vi "Write Element of Coefficients.vi"(8 "error in (no error)":errorcluster, 9 "Numeric":dbl, 10 "index":i32, 11 "Thruster in":refnum<class "Thruster.lvclass">) -> (0 "error out":errorcluster, 3 "Thruster out":refnum<class "Thruster.lvclass">)   [LabVIEW 2014, in "Thruster.lvclass"]
uses:
  Thruster.lvclass
  Thruster.lvclass/Thruster.ctl
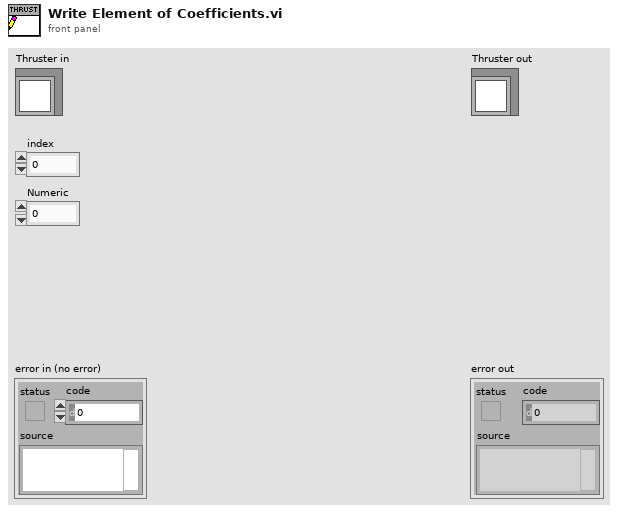
[diagram p1: front panel]
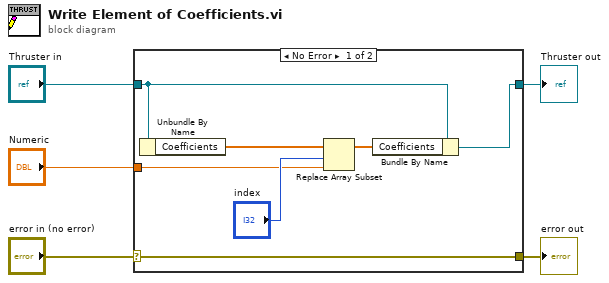
[diagram p0: block diagram]
diagram:
  n1 = case shown="No Error" "error in (no error)" {
    selector: "error in (no error)" -> [w12 w13]
    tunnel: [w12 w13] -> w4
    tunnel: [w11 w14] -> w2
    tunnel: "Thruster in" -> [w10 w14]
    tunnel: "Numeric" -> [w6 _]
    frame No Error {
      n2 = Unbundle By Name(w10) -> ("Coefficients"=w9:dbl[])
      n3 = Replace Array Subset(array=w9, new element=w6, index="index") -> (w8:dbl[])
      n4 = Bundle By Name(cluster=w10, "Coefficients"=w8) -> (w11:refnum<class "Thruster.lvclass">)
    }
    frame Error {
    }
  }
  "error out" <- w4
  "Thruster out" <- w2
